vi "ConvertFDMStringToLVCluster.vi"(1 "FGNetFDM":string) -> (0 "Cluster":T1={"Version"={"version"=20, "pad"=0}, "Positions"={"Doubles"={"longitude"=0.0, "latitude"=0.0, "altitude"=0.0}, "Singles"={"agl"=0.0, "phi"=0.0, "theta"=0.0, "psi"=0.0, "alpha"=0.0, "beta"=0.0}}, "Velocities"={"phidot"=0.0, "thetadot"=0.0, "psidot"=0.0, "vcas"=0.0, "climb_rate"=0.0, "v_north"=0.0, "v_east"=0.0, "v_down"=0.0, "v_wind_body_north"=0.0, "v_wind_body_east"=0.0, "v_wind_body_down"=0.0}, "Accelerations"={"A_X_pilot"=0.0, "A_Y_pilot"=0.0, "A_Z_pilot"=0.0}, "Stall"={"stall_warning"=0.0, "slip_deg"=0.0}, "Engine Status"={"num_engines"=0, "eng_state"=[0, 0, 0, 0], "rpm"=[0.0, 0.0, 0.0, 0.0], "fuel_flow"=[0.0, 0.0, 0.0, 0.0], "fuel_px"=[0.0, 0.0, 0.0, 0.0], "egt"=[0.0, 0.0, 0.0, 0.0], "cht"=[0.0, 0.0, 0.0, 0.0], "mp_osi"=[0.0, 0.0, 0.0, 0.0], "tit"=[0.0, 0.0, 0.0, 0.0], "oil_temp"=[0.0, 0.0, 0.0, 0.0], "oil_px"=[0.0, 0.0, 0.0, 0.0]}, "Consumables"={"num_tanks"=0, "fuel_quantity"=[0.0, 0.0, 0.0, 0.0]}, "Gear Status"={"num_wheels"=0, "wow"=[0, 0, 0, 0], "gear_pos"=[0.0, 0.0, 0.0, 0.0], "gear_steer"=[0.0, 0.0, 0.0, 0.0], "gear_compression"=[0.0, 0.0, 0.0, 0.0]}, "Environment"={"curr_time"=0, "warp"=0, "visibility"=0.0}, "Control Surface Positions"={"elevator"=0.0, "elevator_trim_tab"=0.0, "left_flap"=0.0, "right_flap"=0.0, "left aileron"=0.0, "right_aileron"=0.0, "rudder"=0.0, "nose_wheel"=0.0, "speedbrake"=0.0, "spoilers"=0.0}})   [LabVIEW 2010, in "Flight Gear Data Custom Device.lvlib"]
uses:
  Flight Gear Data Custom Device.lvlib
  FGNetFDM.ctl
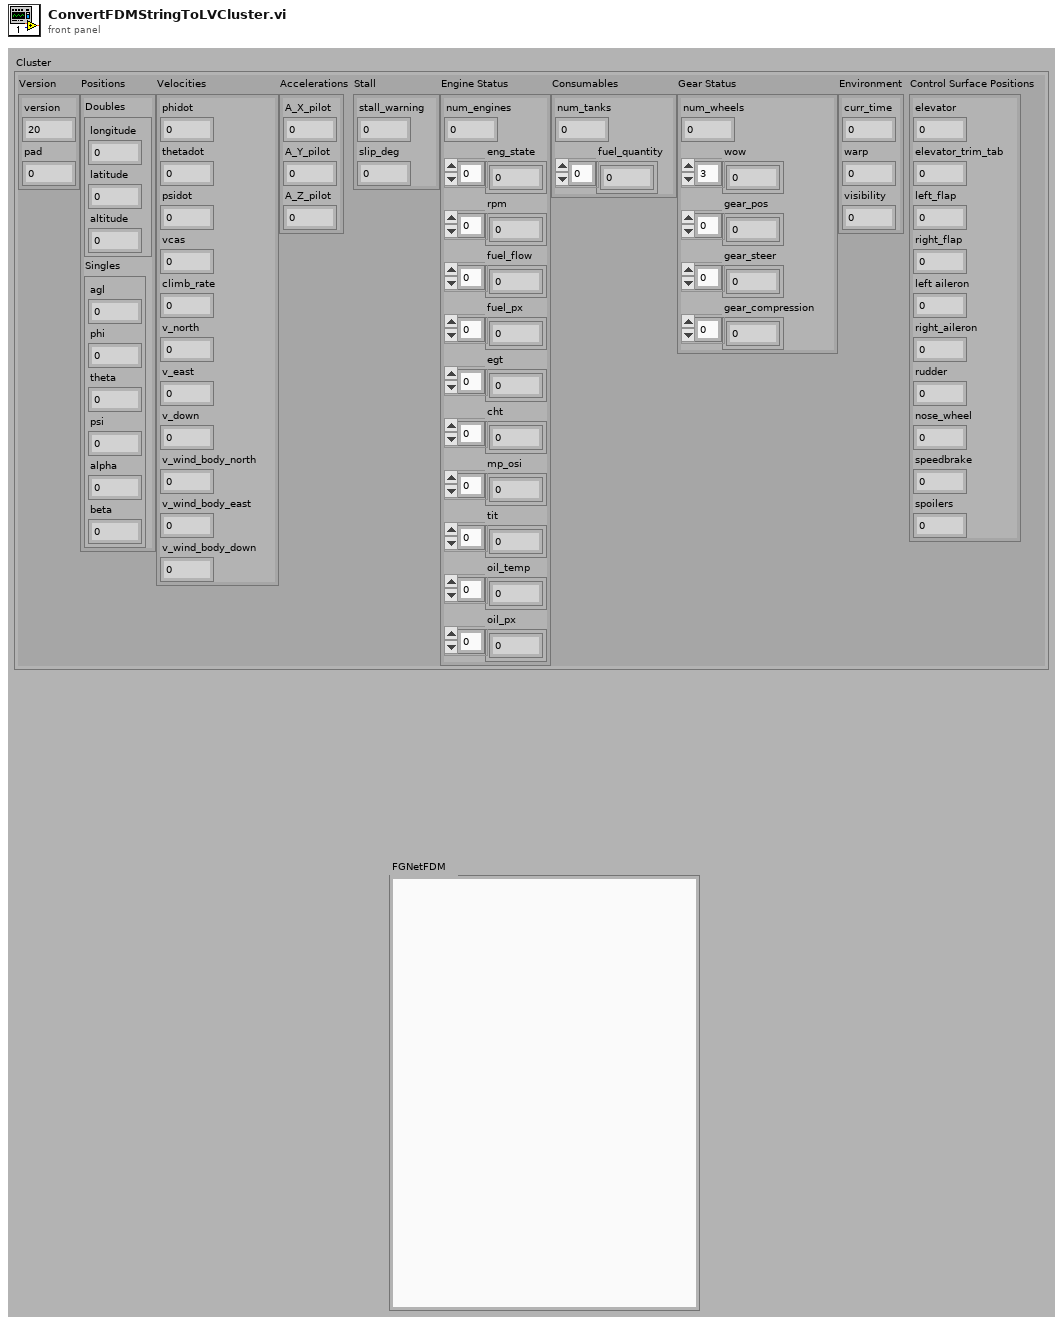
[diagram p1: front panel]
types:
  T1 = typedef "Flight Gear Data Custom Device.lvlib/FGNetFDM.ctl" = cluster{"Version":cluster{"version":u32, "pad":u32}, "Positions":cluster{"Doubles":cluster{"longitude":dbl, "latitude":dbl, "altitude":dbl}, "Singles":cluster{"agl":sgl, "phi":sgl, "theta":sgl, "psi":sgl, "alpha":sgl, "beta":sgl}}, "Velocities":cluster{"phidot":sgl, "thetadot":sgl, "psidot":sgl, "vcas":sgl, "climb_rate":sgl, "v_north":sgl, "v_east":sgl, "v_down":sgl, "v_wind_body_north":sgl, "v_wind_body_east":sgl, "v_wind_body_down":sgl}, "Accelerations":cluster{"A_X_pilot":sgl, "A_Y_pilot":sgl, "A_Z_pilot":sgl}, "Stall":cluster{"stall_warning":sgl, "slip_deg":sgl}, "Engine Status":cluster{"num_engines":u32, "eng_state":u32[], "rpm":sgl[], "fuel_flow":sgl[], "fuel_px":sgl[], "egt":sgl[], "cht":sgl[], "mp_osi":sgl[], "tit":sgl[], "oil_temp":sgl[], "oil_px":sgl[]}, "Consumables":cluster{"num_tanks":u32, "fuel_quantity":sgl[]}, "Gear Status":cluster{"num_wheels":u32, "wow":u32[], "gear_pos":sgl[], "gear_steer":sgl[], "gear_compression":sgl[]}, "Environment":cluster{"curr_time":u32, "warp":i32, "visibility":sgl}, "Control Surface Positions":cluster{"elevator":sgl, "elevator_trim_tab":sgl, "left_flap":sgl, "right_flap":sgl, "left aileron":sgl, "right_aileron":sgl, "rudder":sgl, "nose_wheel":sgl, "speedbrake":sgl, "spoilers":sgl}}
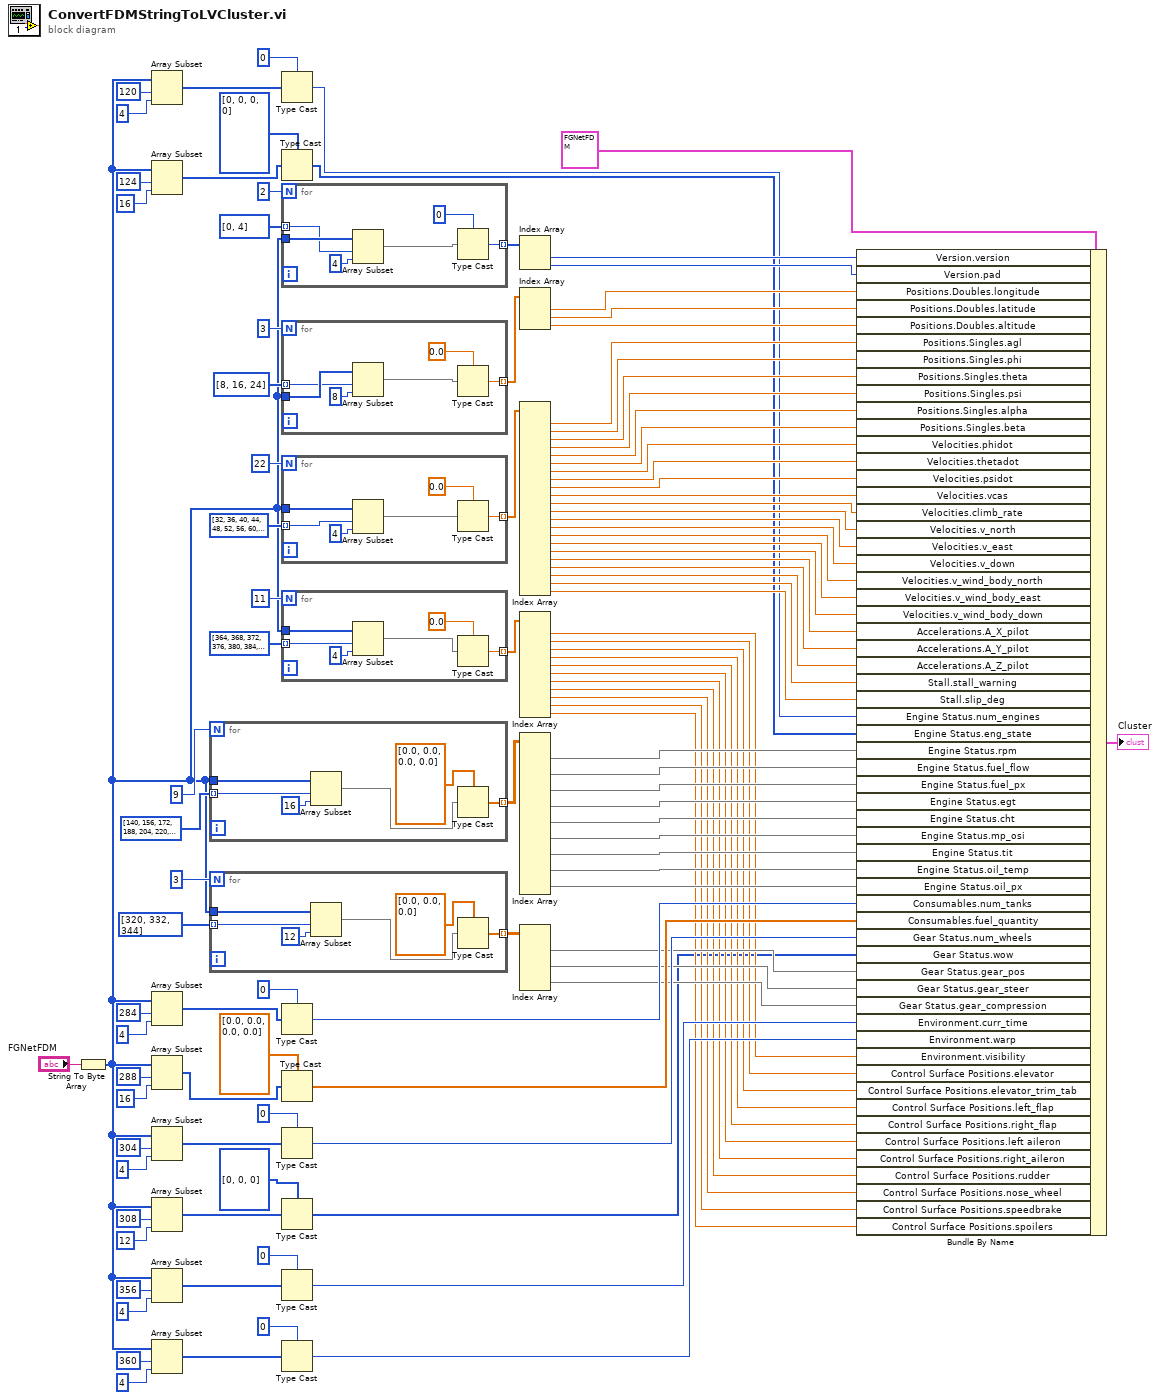
[diagram p0: block diagram]
diagram:
  n1 = String To Byte Array(string="FGNetFDM") -> (unsigned byte array=w2:u8[])
  n2 = Array Subset(array=w2, index=120, length=4) -> (w79:u8[])
  n3 = Array Subset(array=w2, index=124, length=16) -> (w64:u8[])
  n4 = Array Subset(array=w2, index=284, length=4) -> (w61:u8[])
  n5 = Array Subset(array=w2, index=288, length=16) -> (w59:u8[])
  n6 = Array Subset(array=w2, index=304, length=4) -> (w55:u8[])
  n7 = Array Subset(array=w2, index=308, length=12) -> (w27:u8[])
  n8 = Array Subset(array=w2, index=356, length=4) -> (w49:u8[])
  n9 = Array Subset(array=w2, index=360, length=4) -> (w45:u8[])
  n10 = for {
    N: 9 -> [_]
    tunnel: [w116] -> w75 mode=indexing
    tunnel: w2 -> [w118]
    tunnel: i32[] [140, 156, 172, 188, 204, 220, 236, 252, 268] ("Array") -> [w113] mode=indexing
    n11 = Array Subset(array=w118, index=w113, length=16) -> (w117:u8[])
    n12 = Type Cast(type=sgl[] [0.0, 0.0, 0.0, 0.0], x=w117) -> (*(type *) &x=w116:sgl[])
  }
  n13 = for {
    N: 3 -> [_]
    tunnel: [w122] -> w53 mode=indexing
    tunnel: w2 -> [w124]
    tunnel: i32[] [320, 332, 344] ("Array") -> [w119] mode=indexing
    n14 = Array Subset(array=w124, index=w119, length=12) -> (w123:u8[])
    n15 = Type Cast(type=sgl[] [0.0, 0.0, 0.0], x=w123) -> (*(type *) &x=w122:sgl[])
  }
  n16 = Type Cast(type=u32 0 ("length"), x=w79) -> (*(type *) &x=w77:u32)
  n17 = Type Cast(type=u32[] [0, 0, 0, 0], x=w64) -> (*(type *) &x=w74:u32[])
  n18 = for {
    N: 2 -> [_]
    tunnel: [w128] -> w30 mode=indexing
    tunnel: w2 -> [w130]
    tunnel: i32[] [0, 4] -> [w125] mode=indexing
    n19 = Array Subset(array=w130, index=w125, length=4) -> (w127:u8[])
    n20 = Type Cast(type=u32 0 ("length"), x=w127) -> (*(type *) &x=w128:u32)
  }
  n21 = for {
    N: 3 -> [_]
    tunnel: [w134] -> w29 mode=indexing
    tunnel: w2 -> [w136]
    tunnel: i32[] [8, 16, 24] -> [w131] mode=indexing
    n22 = Array Subset(array=w136, index=w131, length=8) -> (w133:u8[])
    n23 = Type Cast(type=0.0 ("length"), x=w133) -> (*(type *) &x=w134:dbl)
  }
  n24 = for {
    N: 22 -> [_]
    tunnel: [w139] -> w28 mode=indexing
    tunnel: w2 -> [w142]
    tunnel: i32[] [32, 36, 40, 44, 48, 52, 56, 60, 64, 68, 72, 76, 80, 84, 88, 92, 96, 100, 104, 108, 112, 116] ("Array") -> [w137] mode=indexing
    n25 = Array Subset(array=w142, index=w137, length=4) -> (w141:u8[])
    n26 = Type Cast(type=sgl 0.0 ("length"), x=w141) -> (*(type *) &x=w139:sgl)
  }
  n27 = for {
    N: 11 -> [_]
    tunnel: [w145] -> w42 mode=indexing
    tunnel: w2 -> [w148]
    tunnel: i32[] [364, 368, 372, 376, 380, 384, 388, 392, 396, 400, 404] ("Array") -> [w143] mode=indexing
    n28 = Array Subset(array=w148, index=w143, length=4) -> (w147:u8[])
    n29 = Type Cast(type=sgl 0.0 ("length"), x=w147) -> (*(type *) &x=w145:sgl)
  }
  n30 = Type Cast(type=u32 0 ("length"), x=w61) -> (*(type *) &x=w60:u32)
  n31 = Type Cast(type=sgl[] [0.0, 0.0, 0.0, 0.0], x=w59) -> (*(type *) &x=w57:sgl[])
  n32 = Type Cast(type=u32 0 ("length"), x=w55) -> (*(type *) &x=w54:u32)
  n33 = Type Cast(type=u32[] [0, 0, 0], x=w27) -> (*(type *) &x=w26:u32[])
  n34 = Type Cast(type=u32 0 ("length"), x=w49) -> (*(type *) &x=w47:u32)
  n35 = Type Cast(type=0 ("length"), x=w45) -> (*(type *) &x=w44:i32)
  n36 = Index Array(array=w30) -> (element #1=w109:u32, element #2=w108:u32)  [unwired: 2 in]
  n37 = Index Array(array=w29) -> (element #1=w106:dbl, element #2=w105:dbl, element #3=w104:dbl)  [unwired: 3 in]
  n38 = Index Array(array=w28) -> (element #1=w102:sgl, element #2=w101:sgl, element #3=w100:sgl, element #4=w99:sgl, element #5=w98:sgl, element #6=w97:sgl, element #7=w96:sgl, element #8=w95:sgl, element #9=w94:sgl, element #10=w93:sgl, element #11=w92:sgl, element #12=w91:sgl, element #13=w90:sgl, element #14=w89:sgl, element #15=w88:sgl, element #16=w87:sgl, element #17=w86:sgl, element #18=w85:sgl, element #19=w84:sgl, element #20=w83:sgl, element #21=w82:sgl, element #22=w81:sgl)  [unwired: 22 in]
  n39 = Index Array(array=w42) -> (element #1=w41:sgl, element #2=w40:sgl, element #3=w39:sgl, element #4=w38:sgl, element #5=w37:sgl, element #6=w36:sgl, element #7=w35:sgl, element #8=w34:sgl, element #9=w33:sgl, element #10=w32:sgl, element #11=w31:sgl)  [unwired: 11 in]
  n40 = Index Array(array=w75) -> (element #1=w73:sgl[], element #2=w72:sgl[], element #3=w71:sgl[], element #4=w70:sgl[], element #5=w69:sgl[], element #6=w68:sgl[], element #7=w67:sgl[], element #8=w66:sgl[], element #9=w65:sgl[])  [unwired: 18 in]
  n41 = Index Array(array=w53) -> (element #1=w52:sgl[], element #2=w51:sgl[], element #3=w50:sgl[])  [unwired: 6 in]
  n42 = Bundle By Name(cluster=T1 {"Version"={"version"=0, "pad"=0}, "Positions"={"Doubles"={"longitude"=0.0, "latitude"=0.0, "altitude"=0.0}, "Singles"={"agl"=0.0, "phi"=0.0, "theta"=0.0, "psi"=0.0, "alpha"=0.0, "beta"=0.0}}, "Velocities"={"phidot"=0.0, "thetadot"=0.0, "psidot"=0.0, "vcas"=0.0, "climb_rate"=0.0, "v_north"=0.0, "v_east"=0.0, "v_down"=0.0, "v_wind_body_north"=0.0, "v_wind_body_east"=0.0, "v_wind_body_down"=0.0}, "Accelerations"={"A_X_pilot"=0.0, "A_Y_pilot"=0.0, "A_Z_pilot"=0.0}, "Stall"={"stall_warning"=0.0, "slip_deg"=0.0}, "Engine Status"={"num_engines"=0, "eng_state"=[], "rpm"=[], "fuel_flow"=[], "fuel_px"=[], "egt"=[], "cht"=[], "mp_osi"=[], "tit"=[], "oil_temp"=[], "oil_px"=[]}, "Consumables"={"num_tanks"=0, "fuel_quantity"=[]}, "Gear Status"={"num_wheels"=0, "wow"=[], "gear_pos"=[], "gear_steer"=[], "gear_compression"=[]}, "Environment"={"curr_time"=0, "warp"=0, "visibility"=0.0}, "Control Surface Positions"={"elevator"=0.0, "elevator_trim_tab"=0.0, "left_flap"=0.0, "right_flap"=0.0, "left aileron"=0.0, "right_aileron"=0.0, "rudder"=0.0, "nose_wheel"=0.0, "speedbrake"=0.0, "spoilers"=0.0}} ("Cluster"), "Version.version"=w109, "Version.pad"=w108, "Positions.Doubles.longitude"=w106, "Positions.Doubles.latitude"=w105, "Positions.Doubles.altitude"=w104, "Positions.Singles.agl"=w102, "Positions.Singles.phi"=w101, "Positions.Singles.theta"=w100, "Positions.Singles.psi"=w99, "Positions.Singles.alpha"=w98, "Positions.Singles.beta"=w97, "Velocities.phidot"=w96, "Velocities.thetadot"=w95, "Velocities.psidot"=w94, "Velocities.vcas"=w93, "Velocities.climb_rate"=w92, "Velocities.v_north"=w91, "Velocities.v_east"=w90, "Velocities.v_down"=w89, "Velocities.v_wind_body_north"=w88, "Velocities.v_wind_body_east"=w87, "Velocities.v_wind_body_down"=w86, "Accelerations.A_X_pilot"=w85, "Accelerations.A_Y_pilot"=w84, "Accelerations.A_Z_pilot"=w83, "Stall.stall_warning"=w82, "Stall.slip_deg"=w81, "Engine Status.num_engines"=w77, "Engine Status.eng_state"=w74, "Engine Status.rpm"=w73, "Engine Status.fuel_flow"=w72, "Engine Status.fuel_px"=w71, "Engine Status.egt"=w70, "Engine Status.cht"=w69, "Engine Status.mp_osi"=w68, "Engine Status.tit"=w67, "Engine Status.oil_temp"=w66, "Engine Status.oil_px"=w65, "Consumables.num_tanks"=w60, "Consumables.fuel_quantity"=w57, "Gear Status.num_wheels"=w54, "Gear Status.wow"=w26, "Gear Status.gear_pos"=w52, "Gear Status.gear_steer"=w51, "Gear Status.gear_compression"=w50, "Environment.curr_time"=w47, "Environment.warp"=w44, "Environment.visibility"=w41, "Control Surface Positions.elevator"=w40, "Control Surface Positions.elevator_trim_tab"=w39, "Control Surface Positions.left_flap"=w38, "Control Surface Positions.right_flap"=w37, "Control Surface Positions.left aileron"=w36, "Control Surface Positions.right_aileron"=w35, "Control Surface Positions.rudder"=w34, "Control Surface Positions.nose_wheel"=w33, "Control Surface Positions.speedbrake"=w32, "Control Surface Positions.spoilers"=w31) -> (→"Cluster":T1)
